vi "Scan Engine Custom FPGA Page - Local.vi"(8 "error in (no error)":errorcluster, 11 "Node Ptr":T1 format="%.0x") -> (0 "error out":errorcluster)   [LabVIEW 2019, in "SEECD System Explorer.lvlib"]
uses:
  SEECD System Explorer.lvlib
  <vilib>/NI VeriStand/Custom Device API/Custom Device Item Ref.ctl
  Type Defs/FPGA Target.ctl
  <vilib>/NI VeriStand/Custom Device API/Custom Device API.lvlib
panel:
  in  "SHDocVw.IWebBrowser2":refnum<k7>(container)
  out "Compilation Target":string
  out "FPGA Bitfile":path caption="Currently Loaded FPGA Personality"
  in  "Clear":bool
  in  "Bitfile Button":bool
  in  "Header":cluster{"Section Name":string}={"Section Name"="Local Chassis Custom FPGA Personality Settings"}
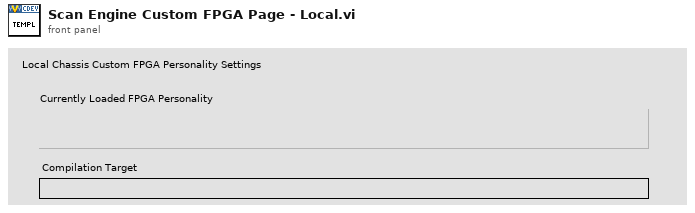
[diagram p1: front panel]
types:
  T1 = typedef "Custom Device API.lvlib/Custom Device Item Ref.ctl" = u64
  T2 = typedef "SEECD System Explorer.lvlib/FPGA Target.ctl" = enum16{"Local", "EtherCAT"}
  T3 = typedef "Custom Device API.lvlib/Custom Device Commands.ctl" = enum16{"Default", "Item renamed", "Shutdown", "Dynamic button pressed"}
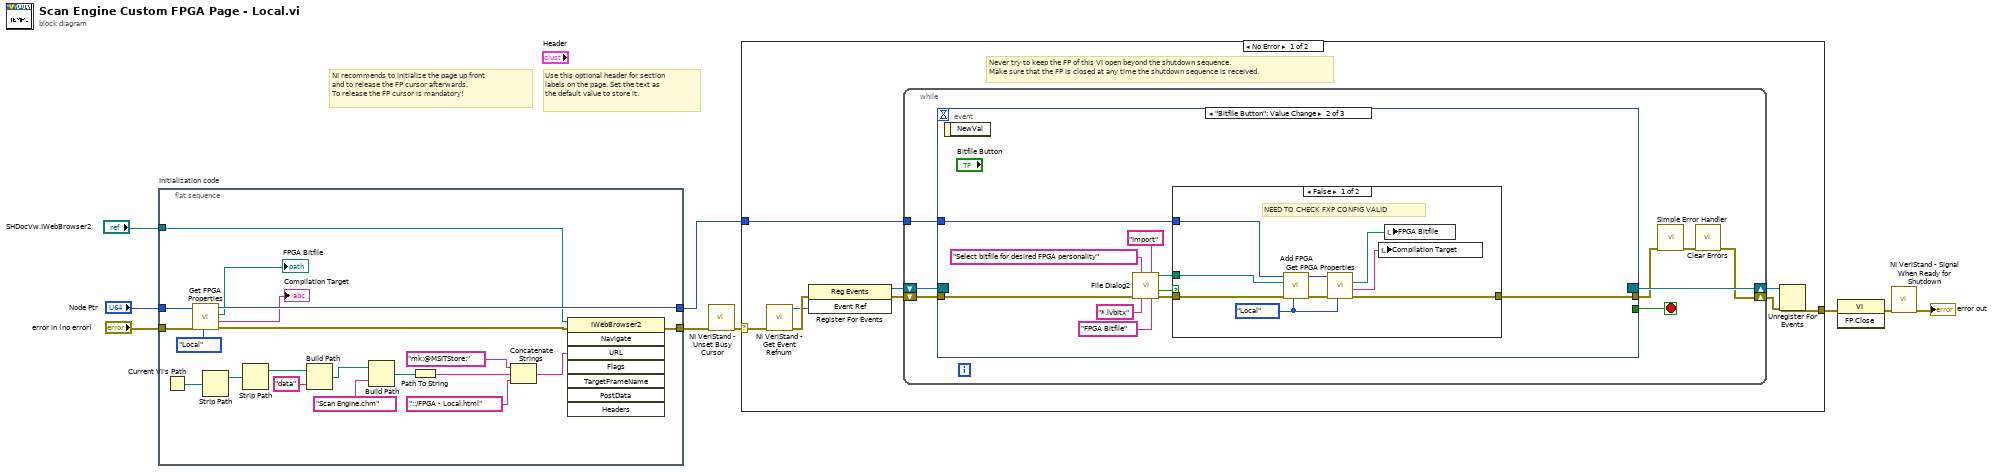
[diagram p0: block diagram]
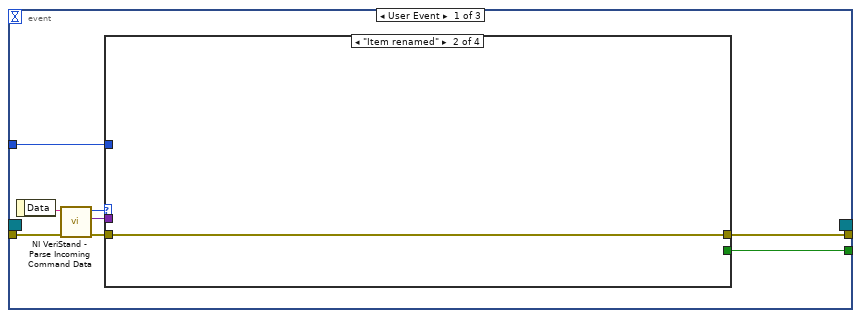
[diagram p2: hidden frame]
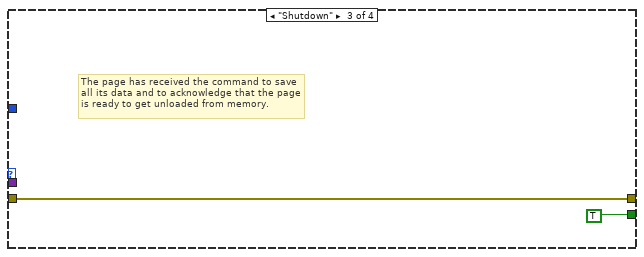
[diagram p4: hidden frame]
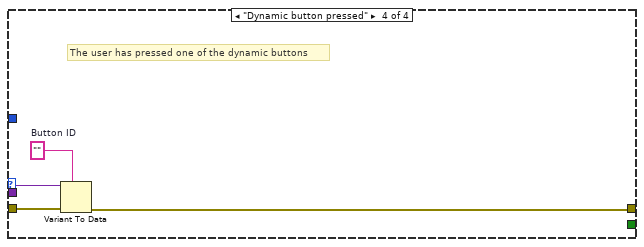
[diagram p5: hidden frame]
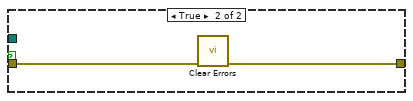
[diagram p6: hidden frame]
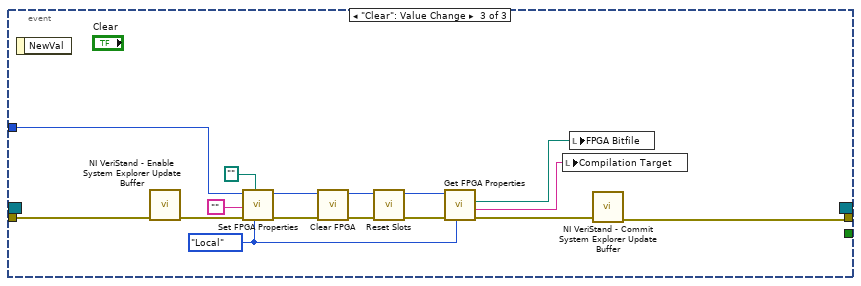
[diagram p7: hidden frame]
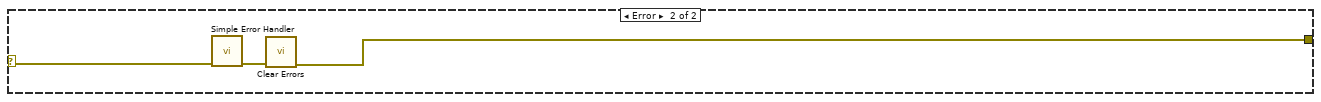
[diagram p8: hidden frame]
diagram:
  # "Use this optional header for section labels on the page. Set the text as the default value to store it."
  # "NI recommends to initialize the page up front\nand to release the FP cursor afterwards.\nTo release the FP cursor is mandatory!"
  n1 = flat-sequence "Initialization code" {
    tunnel: "error in (no error)" -> [w24]
    tunnel: "Node Ptr" -> [w25]
    tunnel: [w13] -> w5
    tunnel: [w29] -> w2
    tunnel: "SHDocVw.IWebBrowser2" -> [w11]
    frame #0 {
      n2 = Current VI's Path() -> (path=w15:path)
      n3 = call "Get FPGA Properties.vi"("FPGA Target"=FPGA_Target."Local", "error in (no error)"=w24, "Item Ref in"=w25) -> ("error out"=w12:errorcluster, "TargetClass"=→"Compilation Target":string, "Bitfile Path"=→"FPGA Bitfile":path, "Item Ref out"=w29:T1)  [unwired: 5 in]
      n4 = Strip Path(path=w15) -> (stripped path=w16:path)  [unwired: 1 out]
      n5 = Strip Path(path=w16) -> (stripped path=w21:path)  [unwired: 1 out]
      n6 = Build Path(base path=w21, name or relative path="data") -> (appended path=w22:path)
      n7 = Build Path(base path=w22, name or relative path="Scan Engine.chm") -> (appended path=w19:path)
      n8 = Path To String(path=w19) -> (string=w18:string)
      n9 = Concatenate Strings("mk:@MSITStore:" ("string"), w18, "::/FPGA - Local.html" ("name or relative path")) -> (w10:string)
      n10 = invoke class="IWebBrowser2" method="Navigate"(reference=w11, error in=w12, "URL"=w10) -> (error out=w13:errorcluster)  [unwired: 5 in, 7 out]
    }
  }
  n11 = call <vilib>:"NI VeriStand - Unset Busy Cursor.vi"("error in (no error)"=w5) -> ("error out"=w4:errorcluster)  [unwired: 10 out]
  n12 = case shown="No Error" w4 {
    selector: w4 -> [w30 w102]
    tunnel: [w35 w100] -> w9
    tunnel: w2 -> [w31 _]
    frame No Error {
      # "Never try to keep the FP of this VI open beyond the shutdown sequence.\nMake sure that the FP is closed at any time the shutdown sequence is received."
      n13 = call <vilib>:"NI VeriStand - Get Event Refnum.vi"("error in (no error)"=w30) -> ("error out"=w38:errorcluster, "Event Ref"=w34:refnum<user-event>)  [unwired: 9 out]
      n14 = register-events(error in=w38, w34) -> (reference out=w32:refnum<event-registration>, error out=w33:errorcluster)  [unwired: 1 in]
      n15 = while {
        tunnel: w31 -> [w42]
        shift-right: [w39] -> w36
        shift-left: w33 -> [w45]
        shift-right: [w46] -> w37
        shift-left: w32 -> [w44]
        stop <- w43 stop-if-true
        n16 = event shown="[1] \"Bitfile Button\": Value Change" {
          selector: w44 -> [_ _ _]
          dyn-events: [_ _ _] -> w46
          timeout: _ -> [_ _ _]
          tunnel: w45 -> [w54 w68 w89]
          tunnel: [w50 _ _] -> w43
          tunnel: [w49 w64 w88] -> w41
          tunnel: w42 -> [w48 w63 w96]
          event User Event {
            n17 = event-data() -> ("Data"=w53:string)  [unwired: 1 out]
            n18 = call <vilib>:"NI VeriStand - Parse Incoming Command Data.vi"("error in (no error)"=w54, "Incoming data"=w53) -> ("error out"=w52:errorcluster, "Outgoing data"=w47:variant, "Action"=w51:T3)  [unwired: 7 out]
            n19 = case shown="\"Item renamed\"" w51 {
              tunnel: w52 -> [w55 w56 w57 w62]
              tunnel: [_ _ TRUE _] -> w50
              tunnel: [w55 w56 w57 w59] -> w49
              tunnel: w48 -> [_ _ _ _]
              tunnel: w47 -> [_ _ _ w61]
              frame "Default", Default {
              }
              frame "Item renamed" {
              }
              frame "Shutdown" {
                # "The page has received the command to save all its data and to acknowledge that the page is ready to get unloaded from memory."
              }
              frame "Dynamic button pressed" {
                w60 = ""  # Button ID
                # "The user has pressed one of the dynamic buttons"
                n20 = Variant To Data(error in=w62, type=w60, Variant=w61) -> (error out=w59:errorcluster)  [unwired: 1 out]
              }
            }
          }
          event "Bitfile Button": Value Change {
            n21 = event-data() -> ()  [unwired: 2 out]
            n22 = call "File Dialog2"("prompt"="Select bitfile for desired FPGA personality", "button label"="Import", "error in"=w68, "pattern (all files)"="*.lvbitx", "pattern label"="FPGA Bitfile") -> ("selected path"=w65:path, "cancelled"=w67:bool, "error out"=w66:errorcluster)  [unwired: 7 in, 1 out]
            n23 = case shown="False" w67 {
              tunnel: w66 -> [w74 w83]
              tunnel: w65 -> [w80 _]
              tunnel: [w73 w82] -> w64
              tunnel: w63 -> [w81 _]
              frame False {
                w77 = FPGA_Target."Local" ("FPGA Target")
                # "NEED TO CHECK FXP CONFIG VALID"
                n24 = call "Add FPGA.vi"("FPGA Target"=w77, "error in (no error)"=w74, "Bitfile Path"=w80, "Item Ref in"=w81) -> ("error out"=w79:errorcluster, "Item Ref out"=w78:T1)  [unwired: 6 in]
                n25 = call "Get FPGA Properties.vi"("FPGA Target"=w77, "error in (no error)"=w79, "Item Ref in"=w78) -> ("error out"=w73:errorcluster, "TargetClass"=w75:string, "Bitfile Path"=w76:path)  [unwired: 5 in, 1 out]
                n26 = local write "Compilation Target"(w75) -> ()
                n27 = local write "FPGA Bitfile"(w76) -> ()
              }
              frame True {
                n28 = call <vilib>:"Clear Errors.vi"("error in (no error)"=w83) -> ("error out"=w82:errorcluster)  [unwired: 1 in, 5 out]
              }
            }
          }
          event "Clear": Value Change {
            w90 = FPGA_Target."Local" ("FPGA Target")
            n29 = event-data() -> ()  [unwired: 2 out]
            n30 = call <vilib>:"NI VeriStand - Enable System Explorer Update Buffer.vi"("error in (no error)"=w89) -> ("error out"=w97:errorcluster)  [unwired: 10 in]
            n31 = call "Set FPGA Properties.vi"("FPGA Target"=w90, "Bitfile Path"=path "", "error in (no error)"=w97, "TargetClass"="", "Item Ref in"=w96) -> ("error out"=w99:errorcluster, "Item Ref out"=w98:T1)  [unwired: 5 in]
            n32 = call "Clear FPGA.vi"("error in (no error)"=w99, "Item Ref in"=w98) -> ("error out"=w87:errorcluster, "Item Ref out"=w86:T1)  [unwired: 8 in]
            n33 = call "Reset Slots.vi"("error in (no error)"=w87, "Item Ref in"=w86) -> ("error out"=w84:errorcluster, "Item Ref out"=w85:T1)  [unwired: 8 in]
            n34 = call "Get FPGA Properties.vi"("FPGA Target"=w90, "error in (no error)"=w84, "Item Ref in"=w85) -> ("error out"=w91:errorcluster, "TargetClass"=w92:string, "Bitfile Path"=w93:path)  [unwired: 5 in, 1 out]
            n35 = local write "Compilation Target"(w92) -> ()
            n36 = local write "FPGA Bitfile"(w93) -> ()
            n37 = call <vilib>:"NI VeriStand - Commit System Explorer Update Buffer.vi"("error in (no error)"=w91) -> ("error out"=w88:errorcluster)  [unwired: 10 in]
          }
        }
        n38 = call <vilib>:"Simple Error Handler.vi"("error in (no error)"=w41) -> ("error out"=w40:errorcluster)  [unwired: 1 in, 7 out]
        n39 = call <vilib>:"Clear Errors.vi"("error in (no error)"=w40) -> ("error out"=w39:errorcluster)  [unwired: 1 in, 5 out]
      }
      n40 = Unregister For Events(event registration refnum=w37, error in=w36) -> (error out=w35:errorcluster)
    }
    frame Error {
      n41 = call <vilib>:"Simple Error Handler.vi"("error in (no error)"=w102) -> ("error out"=w101:errorcluster)  [unwired: 1 in, 7 out]
      n42 = call <vilib>:"Clear Errors.vi"("error in (no error)"=w101) -> ("error out"=w100:errorcluster)  [unwired: 1 in, 5 out]
    }
  }
  n43 = invoke class="VI" method="FP.Close"(error in=w9) -> (error out=w8:errorcluster)  [unwired: 2 in, 2 out]
  n44 = call <vilib>:"NI VeriStand - Signal When Ready for Shutdown.vi"("error in (no error)"=w8) -> ("error out"=→"error out":errorcluster)  [unwired: 10 out]
